vi "Localization.vi"(3 "untranslated":string) -> (1 "translated":string)   [LabVIEW 2023]
doc: "This VI provides human language translations of block diagram strings."
panel:
  in  "translations":string[](array[string])=["Ordered", "Customer failed to pick up item:", "Process Job message dropped!", "#DebugNotification:\nInvalid enqueuer ref when stopping entities."]
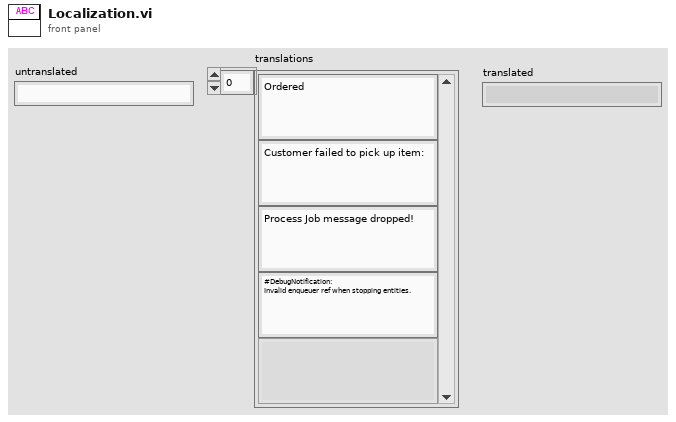
[diagram p1: front panel]
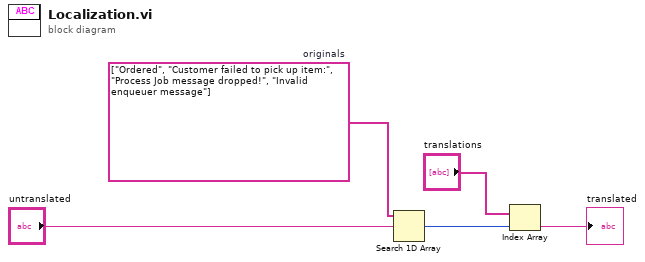
[diagram p0: block diagram]
diagram:
  w5 = string[] ["Ordered", "Customer failed to pick up item:", "Process Job message dropped!", "Invalid enqueuer message"]  # originals
  n1 = Search 1D Array(1D array=w5, element="untranslated") -> (index of element=w2:i32)  [unwired: 1 in]
  n2 = Index Array(array="translations", index=w2) -> (element=→"translated":string)
